vi "GraphForm (SubVI) N.vi"() -> ()   [LabVIEW 2015]
uses:
  Global T.vi
  Global R.vi
panel:
  in  "9_ch_visible":bool=TRUE
  out "T13":dbl format="%.2f"
  out "T11":dbl format="%.2f"
  out "T12":dbl format="%.2f"
  in  "10_ch_visible":bool=TRUE
  in  "11_ch_visible":bool=TRUE
  in  "12_ch_visible":bool=TRUE
  in  "13_ch_visible":bool=TRUE
  in  "14_ch_visible":bool=TRUE
  in  "15_ch_visible":bool=TRUE
  in  "16_ch_visible":bool=TRUE
  in  "1_ch_v":bool=TRUE
  out "T7":dbl format="%.2f"
  out "T5":dbl format="%.2f"
  out "T1":dbl format="%.2f"
  out "T4":dbl format="%.2f"
  in  "R":T1
  in  "stop":bool
  in  "T":T2
  in  "Title":string
  out "часы":string="0"
  in  "Добавить время":dbl(ring)=300.0 items=["1 мин."=60.0, "5 мин."=300.0, "20 мин."=1200.0]
  out "мин.":string="1"
  in  "xScale +":bool
  in  "xScale -":bool
  in  "Autoscale":bool=TRUE
  in  "Т max":u16=300 min=2 max=500 step=1
  in  "Т min":u16=3 min=1 max=350
  in  "2_ch_v":bool=TRUE
  in  "3_ch_v":bool=TRUE
  in  "4_ch_v":bool=TRUE
  in  "5_ch_v":bool=TRUE
  in  "6_ch_v":bool=TRUE
  in  "7_ch_v":bool=TRUE
  in  "8_ch_visible":bool=TRUE
  in  "T7_col":u32(colorbox)=11776947
  in  "T5_col":u32(colorbox)=16711680
  in  "T6_col":u32(colorbox)=6618880
  in  "T3_col":u32(colorbox)=5858815
  in  "T4_col":u32(colorbox)=15688704
  in  "T1_col":u32(colorbox)=16448250
  in  "T2_col":u32(colorbox)=2132224
  out "Graphs T":dynamicdata(graph)
  # "№"
  # "T [К]"
  # "1"
  # "4"
  # "5"
  # "7"
  # "11"
  # "12"
  # "13"
  # "Интервал просмотра"
  # ":"
  # "Шкала Т"
  # "Температура, К"
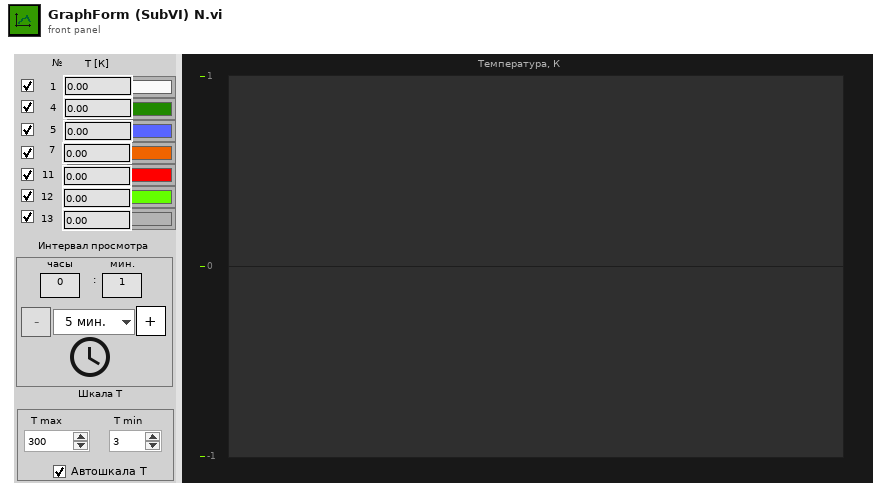
[diagram p1: front panel]
types:
  T1 = cluster{" R1":dbl, " R2":dbl, " R3":dbl, " R4":dbl, " R5":dbl, "R6":dbl, " R7":dbl, "R8":dbl, "R16":dbl, " R15":dbl, "R14":dbl, " R13":dbl, " R12":dbl, " R11":dbl, " R10":dbl, " R9":dbl}
  T2 = cluster{" T1":dbl, " T2":dbl, " T3":dbl, " T4":dbl, " T5":dbl, "T6":dbl, " T7":dbl, "T8":dbl, "T16":dbl, " T15":dbl, "T14":dbl, " T13":dbl, " T12":dbl, " T11":dbl, " T10":dbl, " T9":dbl}
  T3 = cluster{"1":dbl, " 2":dbl, " 3":dbl, "4":dbl, "5":dbl, "6":dbl, "7":dbl, "8":dbl, "9":dbl, " 10":dbl, " 11":dbl, "12":dbl, "13":dbl, "14":dbl, "15":dbl, "16":dbl}
  T4 = cluster{bool, bool, bool, bool, bool, bool, bool, bool, bool, bool, bool, bool, bool, bool, bool, bool}
  T5 = typedef "LVDateTimeRec.ctl" = cluster{"fractional second":dbl, "second":i32, "minute":i32, "hour":i32, "day of month":i32, "month":i32, "year":i32, "day of week":i32, "day of year":i32, "DST":i32}
  T6 = cluster{"1":dbl, " 2":dbl, " 3":dbl, "4":dbl, "5":dbl, "6":dbl, "7":dbl, "8":dbl, "1 2":dbl, " 10":dbl, " 11":dbl, "12":dbl, "13":dbl, "14":dbl, "15":dbl, "16":dbl}
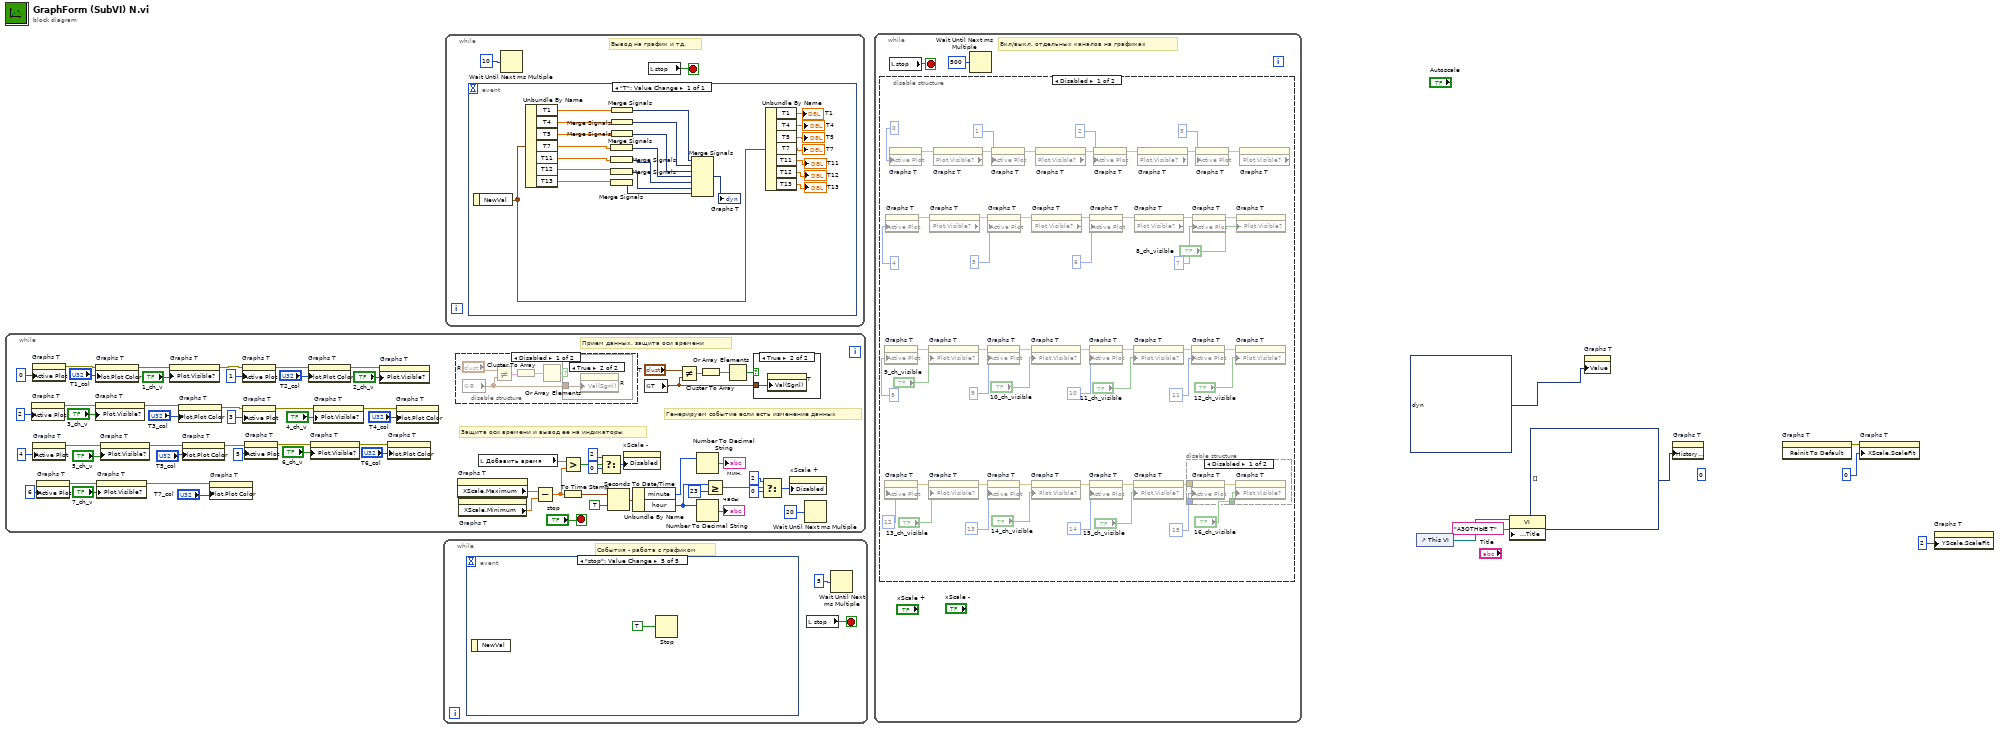
[diagram p0: block diagram]
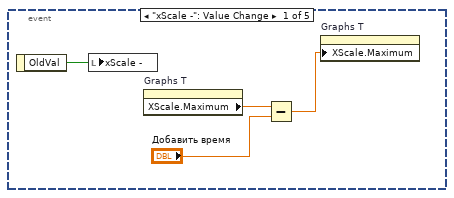
[diagram p7: hidden frame]
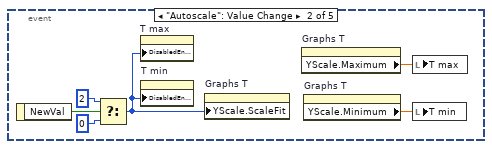
[diagram p8: hidden frame]
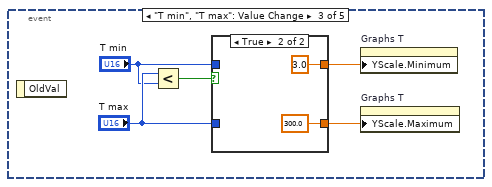
[diagram p9: hidden frame]
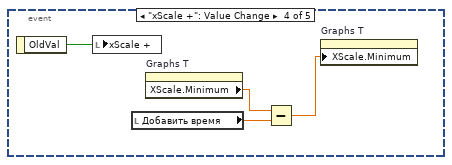
[diagram p11: hidden frame]
diagram:
  (unwired) u8 0 ("Y Scale.Scale Fit")
  n1 = while {
    stop <- "stop" stop-if-true
    # "Генерируем событие если есть изменение данных"
    # "Защита оси времени и вывод ее на индикаторы"
    # "Прием данных, защита оси времени"
    n2 = property on="Graphs T" class="WFChart (strict)"("Active Plot"=u32 2) -> (error out=w18:errorcluster)  [unwired: 2 in, 1 out]
    n3 = property on="Graphs T" class="WFChart (strict)"("Active Plot"=u32 0) -> (error out=w21:errorcluster)  [unwired: 2 in, 1 out]
    n4 = property on="Graphs T" class="WFChart (strict)"("Active Plot"=u32 4) -> (error out=w36:errorcluster)  [unwired: 2 in, 1 out]
    n5 = property on="Graphs T" class="WFChart (strict)"("Active Plot"=u32 6) -> (error out=w34:errorcluster)  [unwired: 2 in, 1 out]
    n6 = property on="Graphs T" class="WFChart (strict)"(error in=w18, "Plot.Visible?"="3_ch_v") -> (error out=w27:errorcluster)  [unwired: 1 in, 1 out]
    n7 = property on="Graphs T" class="WFChart (strict)"(error in=w21, "Plot.Plot Color"="T1_col") -> (error out=w22:errorcluster)  [unwired: 1 in, 1 out]
    n8 = property on="Graphs T" class="WFChart (strict)"(error in=w34, "Plot.Visible?"="7_ch_v") -> (error out=w46:errorcluster)  [unwired: 1 in, 1 out]
    n9 = property on="Graphs T" class="WFChart (strict)"(error in=w36, "Plot.Visible?"="5_ch_v") -> (error out=w38:errorcluster)  [unwired: 1 in, 1 out]
    n10 = property on="Graphs T" class="WFChart (strict)"(error in=w22, "Plot.Visible?"="1_ch_v") -> (error out=w13:errorcluster)  [unwired: 1 in, 1 out]
    n11 = property on="Graphs T" class="WFChart (strict)"(error in=w27, "Plot.Plot Color"="T3_col") -> (error out=w28:errorcluster)  [unwired: 1 in, 1 out]
    n12 = property on="Graphs T" class="WFChart (strict)"(error in=w38, "Plot.Plot Color"="T5_col") -> (error out=w44:errorcluster)  [unwired: 1 in, 1 out]
    n13 = property on="Graphs T" class="WFChart (strict)"(error in=w46, "Plot.Plot Color"="T7_col") -> ()  [unwired: 1 in, 2 out]
    n14 = property on="Graphs T" class="WFChart (strict)"(error in=w13, "Active Plot"=u32 1) -> (error out=w24:errorcluster)  [unwired: 1 in, 1 out]
    n15 = property on="Graphs T" class="WFChart (strict)"(error in=w28, "Active Plot"=u32 3) -> (error out=w17:errorcluster)  [unwired: 1 in, 1 out]
    n16 = property on="Graphs T" class="WFChart (strict)"(error in=w44, "Active Plot"=u32 5) -> (error out=w40:errorcluster)  [unwired: 1 in, 1 out]
    n17 = property on="Graphs T" class="WFChart (strict)"(error in=w24, "Plot.Plot Color"="T2_col") -> (error out=w25:errorcluster)  [unwired: 1 in, 1 out]
    n18 = property on="Graphs T" class="WFChart (strict)"(error in=w40, "Plot.Visible?"="6_ch_v") -> (error out=w42:errorcluster)  [unwired: 1 in, 1 out]
    n19 = property on="Graphs T" class="WFChart (strict)"(error in=w17, "Plot.Visible?"="4_ch_v") -> (error out=w29:errorcluster)  [unwired: 1 in, 1 out]
    n20 = property on="Graphs T" class="WFChart (strict)"(error in=w25, "Plot.Visible?"="2_ch_v") -> ()  [unwired: 1 in, 2 out]
    n21 = property on="Graphs T" class="WFChart (strict)"(error in=w42, "Plot.Plot Color"="T6_col") -> ()  [unwired: 1 in, 2 out]
    n22 = property on="Graphs T" class="WFChart (strict)"(error in=w29, "Plot.Plot Color"="T4_col") -> ()  [unwired: 1 in, 2 out]
    n23 = disable-structure shown="Disabled" {
      frame Disabled {
        n24 = global read "Global R.vi" "R"() -> (w77:T3)
        n25 = Not Equal?(x="R", y=w77) -> (x != y?=w74:T4)
        n26 = Cluster To Array(cluster=w74) -> (array=w75:bool[])
        n27 = Or Array Elements(Boolean array=w75) -> (logical OR=w76:bool)
        n28 = case shown="True" w76 {
          tunnel: w77 -> [_ w78]
          frame False {
          }
          frame True {
            n29 = property on="R" class="Clust (strict)"("Val(Sgnl)"=w78) -> ()  [unwired: 2 in, 2 out]
          }
        }
      }
      frame Enabled {
      }
    }
    n30 = property on="Graphs T" class="WFChart (strict)"() -> ("XScale.Maximum"=w72:dbl)  [unwired: 2 in, 2 out]
    n31 = property on="Graphs T" class="WFChart (strict)"() -> ("XScale.Minimum"=w71:dbl)  [unwired: 2 in, 2 out]
    n32 = local read "Добавить время"() -> (w70:dbl)
    n33 = Subtract(x=w72, y=w71) -> (x-y=w65:dbl)
    n34 = Greater?(x=w70, y=w65) -> (0:w59:bool)
    n35 = To Time Stamp(1:w65) -> (0:w68:timestamp)
    n36 = Select(t=u8 2 ("Disabled"), s=w59, f=u8 0 ("Disabled")) -> (s? t:f=w58:u8)
    n37 = Seconds To Date/Time(time stamp (now)=w68, to UTC (F)=TRUE) -> (date time rec=w67:T5)
    n38 = property on="xScale -" class="Bool (strict)"("Disabled"=w58) -> ()  [unwired: 2 in, 2 out]
    n39 = Unbundle By Name(w67) -> ("minute"=w66:i32, "hour"=w64:i32)
    n40 = global read "Global T.vi" "T"() -> (w47:T6)
    n41 = Not Equal?(x="T", y=w47) -> (x != y?=w51:T4)
    n42 = Number To Decimal String(number=w66) -> (decimal integer string=→"мин.":string)  [unwired: 1 out]
    n43 = Number To Decimal String(number=w64) -> (decimal integer string=→"часы":string)  [unwired: 1 out]
    n44 = Cluster To Array(cluster=w51) -> (array=w50:bool[])
    n45 = Greater Or Equal?(x=w64, y=23) -> (x >= y?=w54:bool)
    n46 = Or Array Elements(Boolean array=w50) -> (logical OR=w49:bool)
    n47 = case shown="True" w49 {
      tunnel: w47 -> [_ w79]
      frame False {
      }
      frame True {
        n48 = property on="T" class="Clust (strict)"("Val(Sgnl)"=w79) -> ()  [unwired: 2 in, 2 out]
      }
    }
    n49 = Select(t=u8 2 ("Disabled"), s=w54, f=u8 0 ("Disabled")) -> (s? t:f=w52:u8)
    n50 = property on="xScale +" class="Bool (strict)"("Disabled"=w52) -> ()  [unwired: 2 in, 2 out]
    n51 = Wait Until Next ms Multiple(millisecond multiple=u32 20) -> ()  [unwired: 1 out]
  }
  n52 = while {
    stop <- w80 stop-if-true
    # "События - работа с графиком"
    n53 = event shown="[4] \"stop\": Value Change" {
      selector: _ -> [_ _ _ _ _]
      dyn-events: _ -> [_ _ _ _ _]
      timeout: _ -> [_ _ _ _ _]
      event "xScale -": Value Change {
        n54 = event-data() -> ("OldVal"=w85:bool)  [unwired: 1 out]
        n55 = local write "xScale -"(w85) -> ()
        n56 = property on="Graphs T" class="WFChart (strict)"() -> ("XScale.Maximum"=w83:dbl)  [unwired: 2 in, 2 out]
        n57 = Subtract(x=w83, y="Добавить время") -> (x-y=w84:dbl)
        n58 = property on="Graphs T" class="WFChart (strict)"("XScale.Maximum"=w84) -> ()  [unwired: 2 in, 2 out]
      }
      event "Autoscale": Value Change {
        n59 = event-data() -> ("NewVal"=w86:bool)  [unwired: 1 out]
        n60 = Select(t=u8 2 ("Y Scale.Scale Fit"), s=w86, f=u8 0 ("Y Scale.Scale Fit")) -> (s? t:f=w89:u8)
        n61 = property on="Т max" class="DigNum (strict)"("DisabledEnum"=w89) -> ()  [unwired: 2 in, 2 out]
        n62 = property on="Т min" class="DigNum (strict)"("DisabledEnum"=w89) -> ()  [unwired: 2 in, 2 out]
        n63 = property on="Graphs T" class="WFChart (strict)"("YScale.ScaleFit"=w89) -> ()  [unwired: 2 in, 2 out]
        n64 = property on="Graphs T" class="WFChart (strict)"() -> ("YScale.Maximum"=w91:dbl)  [unwired: 2 in, 2 out]
        n65 = property on="Graphs T" class="WFChart (strict)"() -> ("YScale.Minimum"=w90:dbl)  [unwired: 2 in, 2 out]
        n66 = local write "Т max"(w91) -> ()
        n67 = local write "Т min"(w90) -> ()
      }
      event "Т min", "Т max": Value Change {
        n68 = event-data() -> ()  [unwired: 2 out]
        n69 = Less?(x="Т max", y="Т min") -> (x < y?=w94:bool)
        n70 = case shown="True" w94 {
          tunnel: [w97 300.0 ("x+1")] -> w96
          tunnel: [w98 3.0 ("x+1")] -> w95
          tunnel: "Т max" -> [w97 _]
          tunnel: "Т min" -> [w98 _]
          frame False {
          }
          frame True {
          }
        }
        n71 = property on="Graphs T" class="WFChart (strict)"("YScale.Minimum"=w95) -> ()  [unwired: 2 in, 2 out]
        n72 = property on="Graphs T" class="WFChart (strict)"("YScale.Maximum"=w96) -> ()  [unwired: 2 in, 2 out]
      }
      event "xScale +": Value Change {
        n73 = event-data() -> ("OldVal"=w104:bool)  [unwired: 1 out]
        n74 = local write "xScale +"(w104) -> ()
        n75 = local read "Добавить время"() -> (w101:dbl)
        n76 = property on="Graphs T" class="WFChart (strict)"() -> ("XScale.Minimum"=w102:dbl)  [unwired: 2 in, 2 out]
        n77 = Subtract(x=w102, y=w101) -> (x-y=w103:dbl)
        n78 = property on="Graphs T" class="WFChart (strict)"("XScale.Minimum"=w103) -> ()  [unwired: 2 in, 2 out]
      }
      event "stop": Value Change {
        n79 = event-data() -> ()  [unwired: 2 out]
        n80 = Stop(stop? (T)=TRUE) -> ()
      }
    }
    n81 = local read "stop"() -> (w80:bool)
    n82 = Wait Until Next ms Multiple(millisecond multiple=u32 5) -> ()  [unwired: 1 out]
  }
  n83 = while {
    stop <- w106 stop-if-true
    # "Вывод на график и тд."
    n84 = event shown="[0] \"T\": Value Change" {
      selector: _ -> [_]
      dyn-events: _ -> [_]
      timeout: _ -> [_]
      event "T": Value Change {
        n85 = event-data() -> ("NewVal"=w123:T2)  [unwired: 1 out]
        n86 = Unbundle By Name(w123) -> ("T1"=w130:dbl, "T4"=w129:dbl, "T5"=w128:dbl, "T7"=w121:dbl, "T11"=w120:dbl, "T12"=w119:dbl, "T13"=w118:dbl)
        n87 = Merge Signals(w121) -> (w117:dynamicdata)
        n88 = Merge Signals(w120) -> (w116:dynamicdata)
        n89 = Merge Signals(w119) -> (w115:dynamicdata)
        n90 = Merge Signals(w118) -> (w114:dynamicdata)
        n91 = Merge Signals(w130) -> (w127:dynamicdata)
        n92 = Merge Signals(w129) -> (w126:dynamicdata)
        n93 = Merge Signals(w128) -> (w125:dynamicdata)
        n94 = Merge Signals(w127, w126, w125, w117, w116, w115, w114) -> (→"Graphs T":dynamicdata)
        n95 = Unbundle By Name(w123) -> ("T1"=→"T1":dbl, "T4"=→"T4":dbl, "T5"=→"T5":dbl, "T7"=→"T7":dbl, "T11"=→"T11":dbl, "T12"=→"T12":dbl, "T13"=→"T13":dbl)
      }
    }
    n96 = Wait Until Next ms Multiple(millisecond multiple=u32 10) -> ()  [unwired: 1 out]
    n97 = local read "stop"() -> (w106:bool)
  }
  n98 = while {
    stop <- w131 stop-if-true
    # "Вкл/выкл. отдельных каналов на графиках"
    n99 = disable-structure shown="Disabled" {
      frame Disabled {
        n100 = property on="Graphs T" class="WFChart (strict)"("Active Plot"=u32 8) -> (error out=w151:errorcluster)  [unwired: 2 in, 1 out]
        n101 = property on="Graphs T" class="WFChart (strict)"("Active Plot"=u32 12) -> (error out=w146:errorcluster)  [unwired: 2 in, 1 out]
        n102 = property on="Graphs T" class="WFChart (strict)"("Active Plot"=u32 4) -> (error out=w187:errorcluster)  [unwired: 2 in, 1 out]
        n103 = property on="Graphs T" class="WFChart (strict)"("Active Plot"=u32 0) -> (error out=w188:errorcluster)  [unwired: 2 in, 1 out]
        n104 = property on="Graphs T" class="WFChart (strict)"(error in=w151, "Plot.Visible?"="9_ch_visible") -> (error out=w153:errorcluster)  [unwired: 1 in, 1 out]
        n105 = property on="Graphs T" class="WFChart (strict)"(error in=w146, "Plot.Visible?"="13_ch_visible") -> (error out=w144:errorcluster)  [unwired: 1 in, 1 out]
        n106 = property on="Graphs T" class="WFChart (strict)"(error in=w187) -> (error out=w185:errorcluster, "Plot.Visible?"=w168:bool)  [unwired: 1 in, 1 out]
        n107 = property on="Graphs T" class="WFChart (strict)"(error in=w188) -> (error out=w190:errorcluster, "Plot.Visible?"=w176:bool)  [unwired: 1 in, 1 out]
        n108 = property on="Graphs T" class="WFChart (strict)"(error in=w153, "Active Plot"=u32 9) -> (error out=w152:errorcluster)  [unwired: 1 in, 1 out]
        n109 = property on="Graphs T" class="WFChart (strict)"(error in=w144, "Active Plot"=u32 13) -> (error out=w145:errorcluster)  [unwired: 1 in, 1 out]
        n110 = property on="Graphs T" class="WFChart (strict)"(error in=w185, "Active Plot"=u32 5) -> (error out=w186:errorcluster)  [unwired: 1 in, 1 out]
        n111 = property on="Graphs T" class="WFChart (strict)"(error in=w190, "Active Plot"=u32 1) -> (error out=w189:errorcluster)  [unwired: 1 in, 1 out]
        n112 = property on="Graphs T" class="WFChart (strict)"(error in=w152, "Plot.Visible?"="10_ch_visible") -> (error out=w155:errorcluster)  [unwired: 1 in, 1 out]
        n113 = property on="Graphs T" class="WFChart (strict)"(error in=w145, "Plot.Visible?"="14_ch_visible") -> (error out=w142:errorcluster)  [unwired: 1 in, 1 out]
        n114 = property on="Graphs T" class="WFChart (strict)"(error in=w186) -> (error out=w183:errorcluster, "Plot.Visible?"=w166:bool)  [unwired: 1 in, 1 out]
        n115 = property on="Graphs T" class="WFChart (strict)"(error in=w189) -> (error out=w191:errorcluster, "Plot.Visible?"=w174:bool)  [unwired: 1 in, 1 out]
        n116 = property on="Graphs T" class="WFChart (strict)"(error in=w155, "Active Plot"=u32 10) -> (error out=w154:errorcluster)  [unwired: 1 in, 1 out]
        n117 = property on="Graphs T" class="WFChart (strict)"(error in=w142, "Active Plot"=u32 14) -> (error out=w143:errorcluster)  [unwired: 1 in, 1 out]
        n118 = property on="Graphs T" class="WFChart (strict)"(error in=w183, "Active Plot"=u32 6) -> (error out=w184:errorcluster)  [unwired: 1 in, 1 out]
        n119 = property on="Graphs T" class="WFChart (strict)"(error in=w191, "Active Plot"=u32 2) -> (error out=w178:errorcluster)  [unwired: 1 in, 1 out]
        n120 = property on="Graphs T" class="WFChart (strict)"(error in=w154, "Plot.Visible?"="11_ch_visible") -> (error out=w157:errorcluster)  [unwired: 1 in, 1 out]
        n121 = property on="Graphs T" class="WFChart (strict)"(error in=w143, "Plot.Visible?"="15_ch_visible") -> (error out=w141:errorcluster)  [unwired: 1 in, 1 out]
        n122 = property on="Graphs T" class="WFChart (strict)"(error in=w184) -> (error out=w181:errorcluster, "Plot.Visible?"=w164:bool)  [unwired: 1 in, 1 out]
        n123 = property on="Graphs T" class="WFChart (strict)"(error in=w178) -> (error out=w179:errorcluster, "Plot.Visible?"=w172:bool)  [unwired: 1 in, 1 out]
        n124 = disable-structure shown="Disabled" {
          disable-tunnel: w141 -> [w194 _]
          disable-tunnel: u32 15 ("Active Plot") -> [w193 _]
          disable-tunnel: "16_ch_visible" -> [w192 _]
          frame Disabled {
            n125 = property on="Graphs T" class="WFChart (strict)"(error in=w194, "Active Plot"=w193) -> (error out=w195:errorcluster)  [unwired: 1 in, 1 out]
            n126 = property on="Graphs T" class="WFChart (strict)"(error in=w195, "Plot.Visible?"=w192) -> ()  [unwired: 1 in, 2 out]
          }
          frame Enabled {
          }
        }
        n127 = property on="Graphs T" class="WFChart (strict)"(error in=w157, "Active Plot"=u32 11) -> (error out=w156:errorcluster)  [unwired: 1 in, 1 out]
        n128 = property on="Graphs T" class="WFChart (strict)"(error in=w181, "Active Plot"=u32 7) -> (error out=w182:errorcluster)  [unwired: 1 in, 1 out]
        n129 = property on="Graphs T" class="WFChart (strict)"(error in=w179, "Active Plot"=u32 3) -> (error out=w180:errorcluster)  [unwired: 1 in, 1 out]
        n130 = property on="Graphs T" class="WFChart (strict)"(error in=w156, "Plot.Visible?"="12_ch_visible") -> ()  [unwired: 1 in, 2 out]
        n131 = property on="Graphs T" class="WFChart (strict)"(error in=w182, "Plot.Visible?"="8_ch_visible") -> ()  [unwired: 1 in, 2 out]
        n132 = property on="Graphs T" class="WFChart (strict)"(error in=w180) -> ("Plot.Visible?"=w170:bool)  [unwired: 1 in, 2 out]
      }
      frame Enabled {
      }
    }
    n133 = local read "stop"() -> (w131:bool)
    n134 = Wait Until Next ms Multiple(millisecond multiple=u32 500) -> ()  [unwired: 1 out]
  }
  n135 = control-ref of="This VI"() -> (w2:refnum<vi>)
  n136 = property class="VI"(reference=w2, "Front Panel.Title"="АЗОТНЫЕ Т" ("Front Panel Window:Title")) -> ()  [unwired: 1 in, 2 out]
  n137 = property on="Graphs T" class="WFChart (strict)"("Value"=dynamicdata [{"t0"=timestamp(3465273261.7246556 s since 1904-01-01), "dt"=1.0, "Y"=[0.1931097262457384]}, {"t0"=timestamp(3465273261.7246556 s since 1904-01-01), "dt"=1.0, "Y"=[0.3594116459482981]}, {"t0"=timestamp(3465273261.7246556 s since 1904-01-01), "dt"=1.0, "Y"=[0.8898205452798131]}, {"t0"=timestamp(3465273261.7246556 s since 1904-01-01), "dt"=1.0, "Y"=[0.747699236883661]}] ("Graphs")) -> ()  [unwired: 2 in, 2 out]
  n138 = property on="Graphs T" class="WFChart (strict)"("History Data"=dynamicdata[] []) -> ()  [unwired: 2 in, 2 out]
  n139 = invoke on="Graphs T" class="WFChart (strict)" method="Reinit To Default"() -> (error out=w4:errorcluster)  [unwired: 3 in, 2 out]
  n140 = property on="Graphs T" class="WFChart (strict)"(error in=w4, "XScale.ScaleFit"=u8 0 ("Y Scale.Scale Fit")) -> ()  [unwired: 1 in, 2 out]
  n141 = property on="Graphs T" class="WFChart (strict)"("YScale.ScaleFit"=u8 2 ("Y Scale.Scale Fit")) -> ()  [unwired: 2 in, 2 out]
